vi "Export Groups.vi"(8 "error in (no error)":errorcluster, 10 "Path":path, 11 "BluelinesRedlines in":refnum<class "BluelinesRedlines.lvclass">) -> (0 "error out":errorcluster, 3 "BluelinesRedlines out":refnum<class "BluelinesRedlines.lvclass">)   [LabVIEW 2023, in "VolatusGUIElements.lvlib" / "BluelinesRedlines.lvclass"]
uses:
  BluelinesRedlines.lvclass
  BluelinesRedlines.lvclass/BluelinesRedlines.ctl
  User BluelinesRedlines/User BluelinesRedlines.lvclass
  lv-cdm/CDM-Config/Config-JSON/Config-JSON.lvclass
  C:/dev/volatus/mts-volatus-super/libs/lv-cdm/CDM-Config/Config Storage/Config Storage.lvclass
  lv-cdm/CDM-Config/Config Element/Write Variant Value.vi
  lv-cdm/CDM-Config/Config Manager/Config Manager.lvclass
  lv-cdm/CDM-Config/Config Element/Config Element.lvclass
  lv-cdm/CDM-Config/Config Storage/Config Storage.lvclass
  C:/dev/volatus/mts-volatus-super/libs/lv-cdm/CDM-Config/Config-JSON/Config-JSON.lvclass
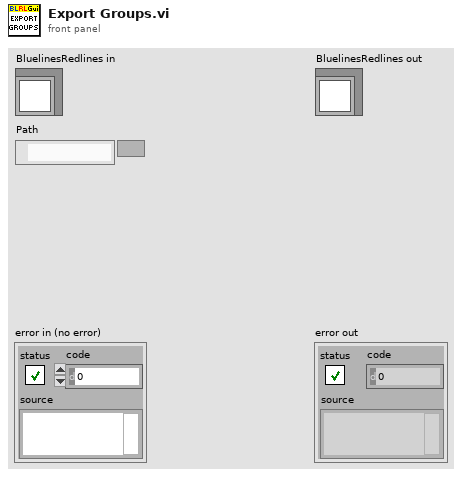
[diagram p1: front panel]
types:
  T1 = map{string, refnum<class "BluelinesRedlines Source.lvclass">}
  T2 = typedef "VolatusGUI.lvlib/BluelinesRedlines Source.lvclass/BLRL Config.ctl" = cluster{"Bluelines":T3[], "Redlines":T3[]}
  T3 = typedef "VolatusGUI.lvlib/BluelinesRedlines Source.lvclass/Range Limit Config.ctl" = cluster{"Channel":string, "Low Limit":dbl, "High Limit":dbl}
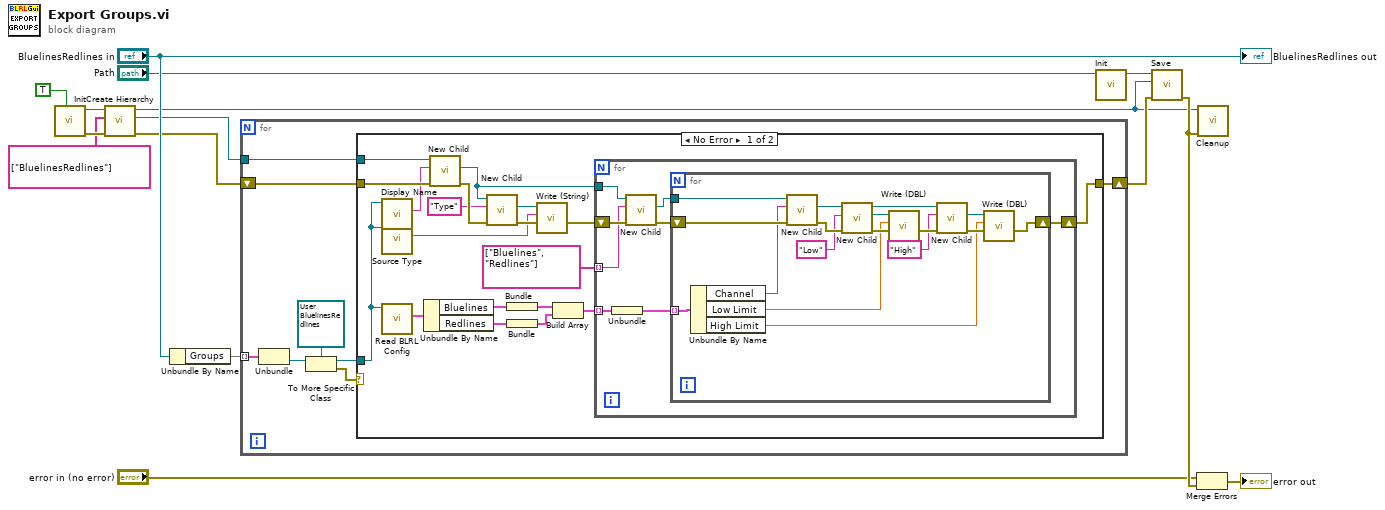
[diagram p0: block diagram]
diagram:
  n1 = call "Init.vi"("Unlock Writes (F)"=TRUE) -> ("error out"=w12:errorcluster, "Config Manager out"=w11:refnum<class "Config Manager.lvclass">)  [unwired: 9 in]
  n2 = call "Create Hierarchy.vi"("error in (no error)"=w12, "Hierarchy"=string[] ["BluelinesRedlines"], "Config Manager in"=w11) -> ("error out"=w9:errorcluster, "Leaf Element"=w8:refnum<class "Config Element.lvclass">, "Config Manager out"=w2:refnum<class "Config Manager.lvclass">)  [unwired: 6 in]
  n3 = Unbundle By Name("BluelinesRedlines in") -> ("Groups"=w13:T1)
  n4 = for {
    tunnel: w13 -> [w23] mode=indexing
    shift-right: [w16] -> w5
    shift-left: w9 -> [w17]
    tunnel: w8 -> [w18]
    n5 = Unbundle(w23) -> ("VolatusGUI:BluelinesRedlines Source.lvclass"=w22:refnum<class "BluelinesRedlines Source.lvclass">)  [unwired: 1 out]
    n6 = To More Specific Class(target class=refnum<class "User BluelinesRedlines.lvclass"> refnum ("VolatusGUIElements.lvlib:User BluelinesRedlines.lvclass"), reference=w22) -> (specific class reference=w19:refnum<class "User BluelinesRedlines.lvclass">, error out=w20:errorcluster)  [unwired: 1 in]
    n7 = case shown="No Error" w20 {
      tunnel: w19 -> [w34 _]
      tunnel: w18 -> [w42 _]
      tunnel: w17 -> [w41 w68]
      tunnel: [w24 w68] -> w16
      frame No Error {
        n8 = call-dynamic "Display Name.vi"("User BluelinesRedlines in"=w34) -> ("Display Name"=w40:string)  [unwired: 10 in]
        n9 = call-dynamic "Source Type.vi"("User BluelinesRedlines in"=w34) -> ("Source Type"=w35:string)  [unwired: 10 in]
        n10 = call-dynamic "Read BLRL Config.vi"("User BluelinesRedlines in"=w34) -> ("BLRL Config"=w33:T2)  [unwired: 8 in, 2 out]
        n11 = Unbundle By Name(w33) -> ("Bluelines"=w32:T3[], "Redlines"=w31:T3[])
        n12 = call "New Child.vi"("error in (no error)"=w41, "Child Name"=w40, "Config Element in"=w42) -> ("error out"=w39:errorcluster, "New Child"=w27:refnum<class "Config Element.lvclass">)  [unwired: 6 in, 1 out]
        n13 = call "New Child.vi"("error in (no error)"=w39, "Child Name"="Type", "Config Element in"=w27) -> ("error out"=w37:errorcluster, "New Child"=w36:refnum<class "Config Element.lvclass">)  [unwired: 6 in, 1 out]
        n14 = Bundle("Bluelines"=w32) -> (w30:cluster{"Bluelines":T3[]})  [unwired: 1 in]
        n15 = Bundle("Redlines"=w31) -> (w29:cluster{"Redlines":T3[]})  [unwired: 1 in]
        n16 = call "Write (String).vi"("error in (no error)"=w37, "String Value"=w35, "Config Element in"=w36) -> ("error out"=w26:errorcluster)  [unwired: 7 in, 1 out]
        n17 = Build Array(w30, w29) -> (w28:cluster{"Redlines":T3[]}[])
        n18 = for {
          tunnel: w28 -> [w47] mode=indexing
          tunnel: w27 -> [w49]
          shift-right: [w43] -> w24
          shift-left: w26 -> [w50]
          tunnel: string[] ["Bluelines", "Redlines"] -> [w48] mode=indexing
          n19 = Unbundle(w47) -> ("Redlines"=w44:T3[])
          n20 = call "New Child.vi"("error in (no error)"=w50, "Child Name"=w48, "Config Element in"=w49) -> ("error out"=w46:errorcluster, "New Child"=w45:refnum<class "Config Element.lvclass">)  [unwired: 6 in, 1 out]
          n21 = for {
            shift-right: [w51] -> w43
            shift-left: w46 -> [w67]
            tunnel: w45 -> [w66]
            tunnel: w44 -> [w65] mode=indexing
            n22 = Unbundle By Name(w65) -> ("Channel"=w64:string, "Low Limit"=w58:dbl, "High Limit"=w52:dbl)
            n23 = call "New Child.vi"("error in (no error)"=w67, "Child Name"=w64, "Config Element in"=w66) -> ("error out"=w62:errorcluster, "New Child"=w63:refnum<class "Config Element.lvclass">)  [unwired: 6 in, 1 out]
            n24 = call "New Child.vi"("error in (no error)"=w62, "Child Name"="Low", "Config Element in"=w63) -> ("error out"=w60:errorcluster, "New Child"=w59:refnum<class "Config Element.lvclass">, "Config Element out"=w54:refnum<class "Config Element.lvclass">)  [unwired: 6 in]
            n25 = call "Write (DBL).vi"("error in (no error)"=w60, "DBL Value"=w58, "Config Element in"=w59) -> ("error out"=w55:errorcluster)  [unwired: 7 in, 1 out]
            n26 = call "New Child.vi"("error in (no error)"=w55, "Child Name"="High", "Config Element in"=w54) -> ("error out"=w56:errorcluster, "New Child"=w57:refnum<class "Config Element.lvclass">)  [unwired: 6 in, 1 out]
            n27 = call "Write (DBL).vi"("error in (no error)"=w56, "DBL Value"=w52, "Config Element in"=w57) -> ("error out"=w51:errorcluster)  [unwired: 7 in, 1 out]
          }
        }
      }
      frame Error {
        # "Not a User defined group, do not export."
      }
    }
  }
  n28 = call "Init.vi"("Path"="Path") -> ("Config-JSON out"=w6:refnum<class "Config-JSON.lvclass">)  [unwired: 9 in, 1 out]
  n29 = call "Save.vi"("error in (no error)"=w5, "Config"=w2, "Config Storage in"=w6) -> ("error out"=w15:errorcluster)  [unwired: 7 in, 1 out]
  n30 = Merge Errors("error in (no error)", w15) -> (→"error out":errorcluster)
  n31 = call "Cleanup.vi"("error in (no error)"=w15, "Config Manager in"=w2) -> ()  [unwired: 9 in, 1 out]
  "BluelinesRedlines out" <- "BluelinesRedlines in"
